vi "LSCI_6-19.vi"() -> ()   [LabVIEW 2019]
uses:
  Control 2.ctl
  Settings.ctl
  <vilib>/DAQmx/write.llb/DAQmx Write (Analog 1D DBL 1Chan NSamp).vi
  <vilib>/DAQmx/create/channels.llb/DAQmx Create Channel (AO-Voltage-Basic).vi
  <vilib>/DAQmx/configure/timing.llb/DAQmx Timing (Sample Clock).vi
  <vilib>/DAQmx/miscellaneous.llb/DAQmx Fill In Error Info.vi
panel:
  out "LSCI Sequence 2":dbl[](graph)
  in  "Stop":bool
  in  "Strength (V)":dbl=5.0
  in  "Width of pulse (ms)":dbl=70.0
  in  "Delay End (ms)":i32=52
  in  "Delay (ms)":dbl=20.0
  in  "AOM Voltage":dbl=0.135 format="%0.3f"
  out "String 7":string="AOM Settings"
  out "String 6":string="Stroke Settings"
  out "String 5":string="Intrinsic Imaging"
  in  "LED 625 nm":bool
  in  "LED 580 nm":bool
  out "Period (ms)":dbl=6.0
  out "String 4":string="Experimental Summary"
  out "String 3":string="Stimulation Control"
  out "String 2":string="Sequence Control"
  out "String":string="Trials Control"
  in  "Strength (V)":dbl=5.0
  in  "# of stimulations":i32=20
  in  "Delay (ms)":dbl=20.0
  in  "Width of pulse (ms)":dbl=70.0
  in  "# of Sequences":dbl=300.0
  in  "Delay End (ms)":i32=52
  in  "Sampling Rate (Hz)":T1=100000.0 format="%#_9f"
  in  "Frames/Seq":i32=8
  in  "Exposure Width (ms)":T1=5.0 format="%#_9f"
  in  "Time Between (ms)":T2=1.0 format="%#_9f"
  in  "Pre-stimulus Time":dbl=2.5 format="%.6f"
  in  "Time b/w Trials (s)":dbl=20.0 caption="Delay Time (s)"
  in  "# Trials":i32=50
  in  "Time domain signal":enum32{"Trigger Sequence", "Stimulation pulse"}(tab)
  out "LSCI Sequence":cluster{i32, dbl, dbl[]}(graph)={0, 1e-05, array[10000 elements]}
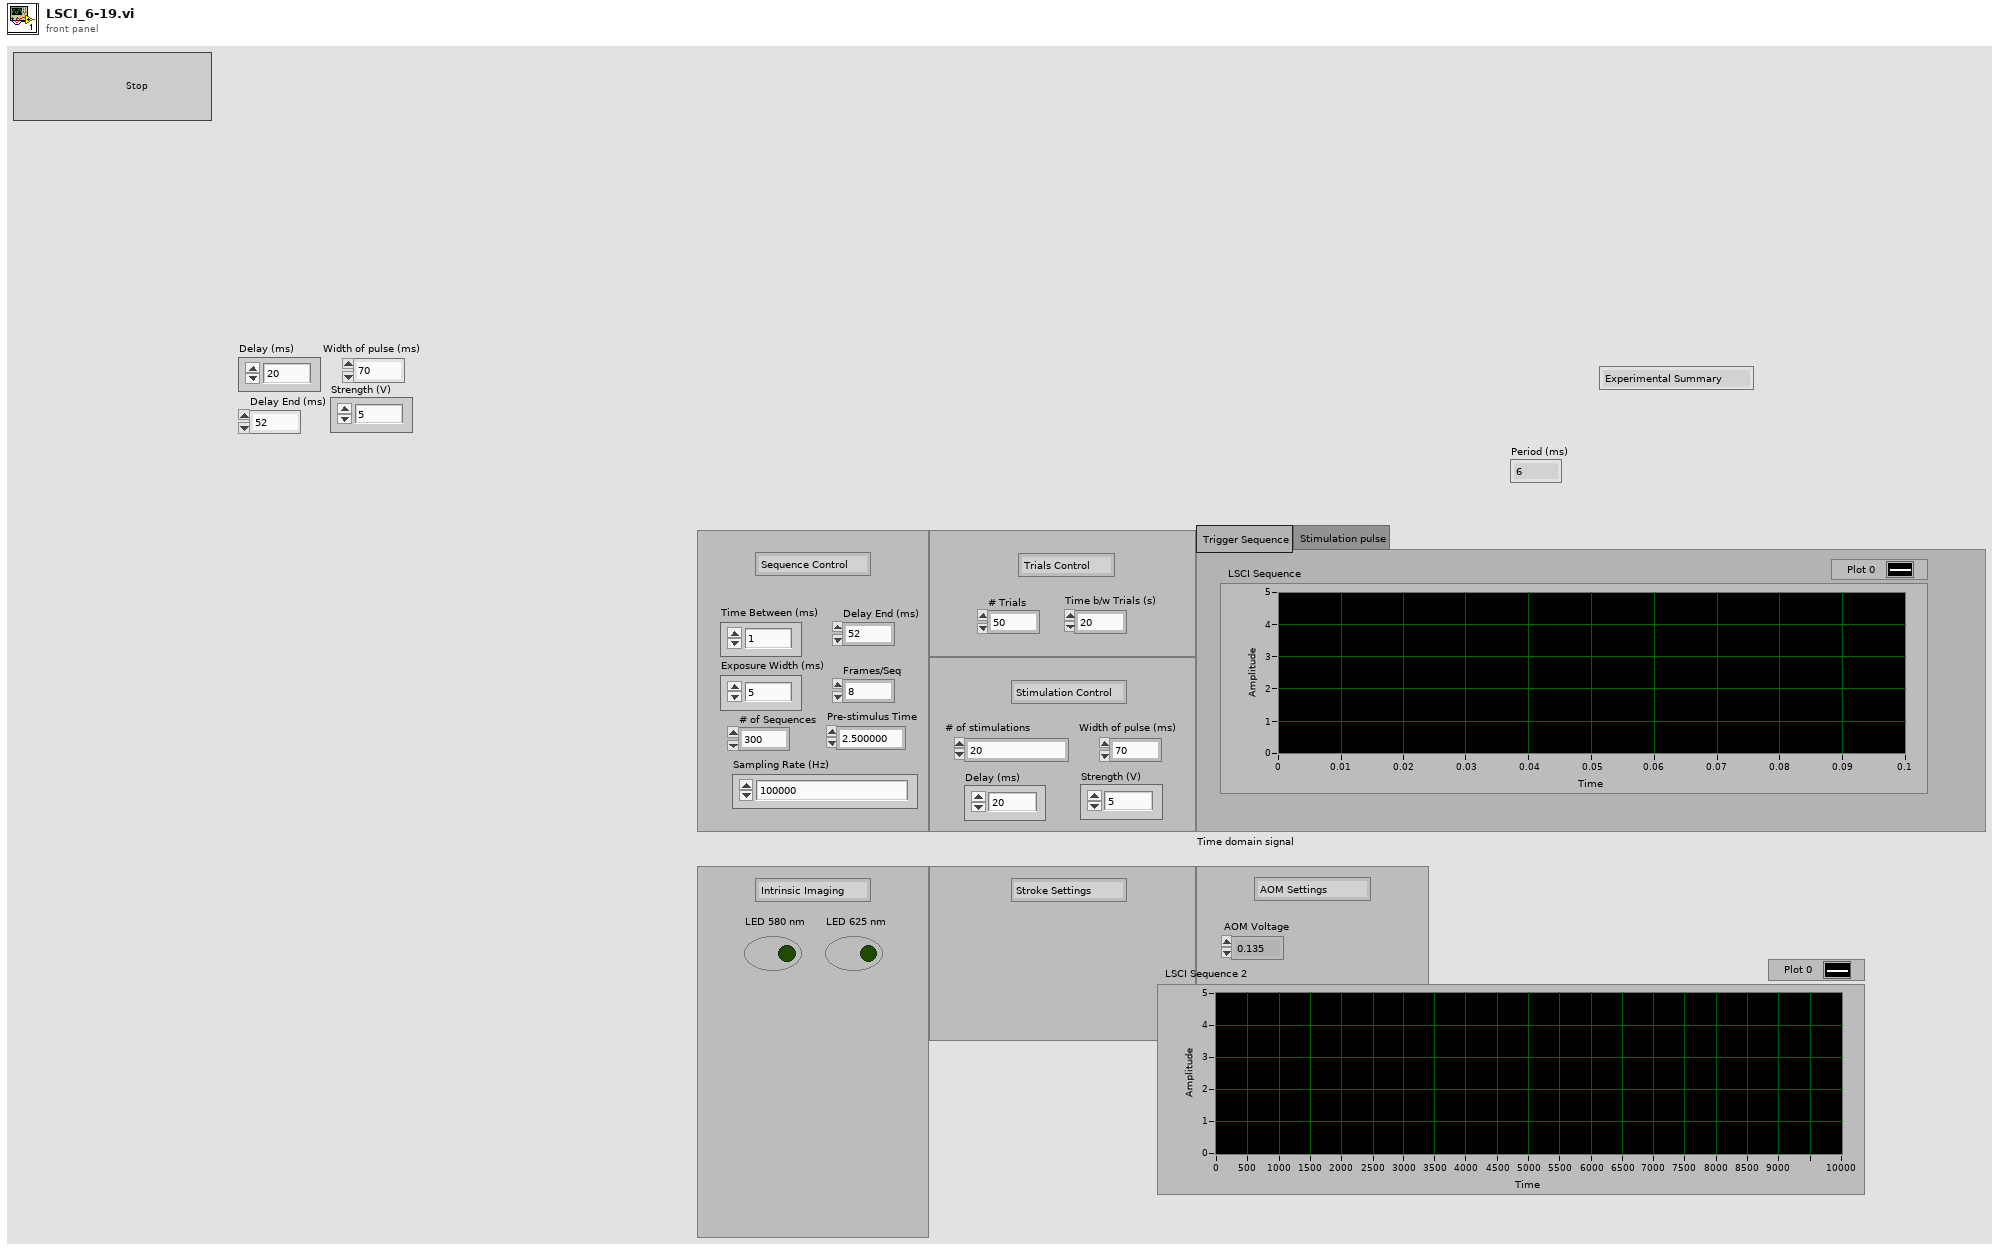
[diagram p1: front panel]
types:
  T1 = typedef "Settings.ctl" = dbl
  T2 = typedef "Control 2.ctl" = dbl
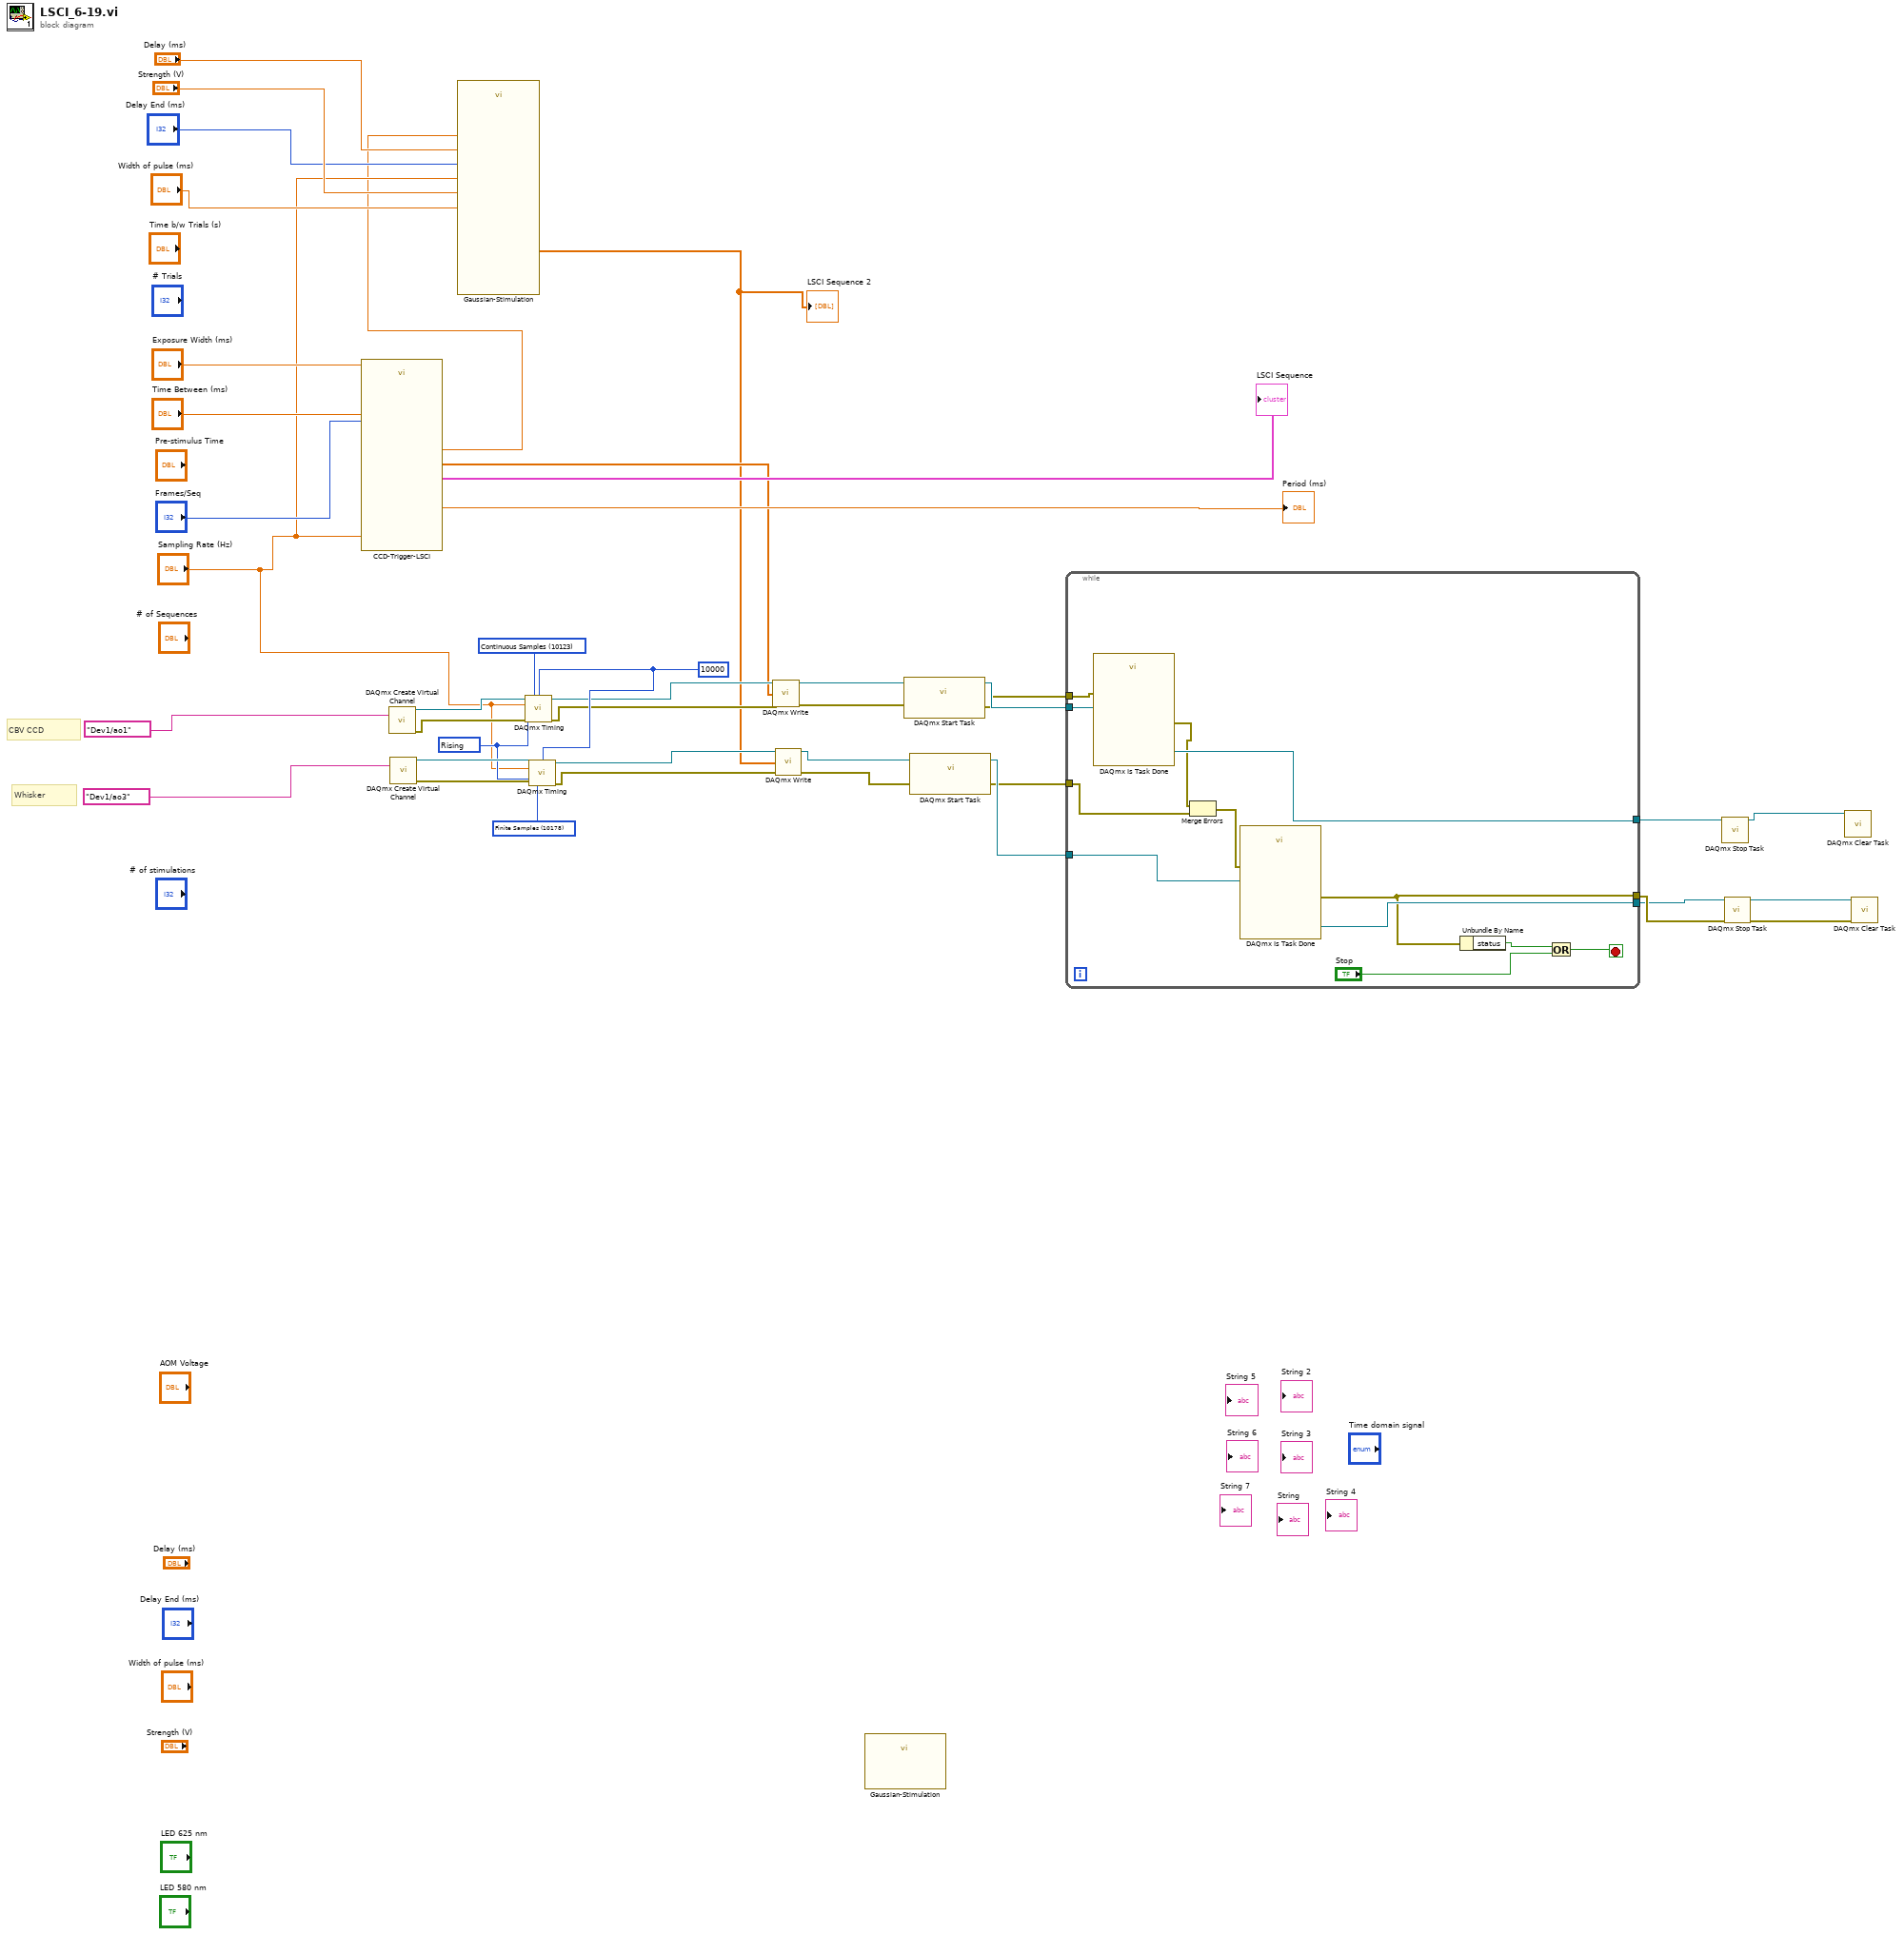
[diagram p0: block diagram]
diagram:
  w28 = 10178 items=["Finite Samples"=10178, "Continuous Samples"=10123, "Hardware Timed Single Point"=12522] ("sample mode")
  w27 = 10000 ("samples per channel")
  w32 = 10123 items=["Finite Samples"=10178, "Continuous Samples"=10123, "Hardware Timed Single Point"=12522] ("sample mode")
  w29 = 10280 items=["Rising"=10280, "Falling"=10171] ("active edge")
  # "CBV CCD"
  # "Whisker"
  n1 = call "CCD-Trigger-LSCI.vi"("Sampling Rate"="Sampling Rate (Hz)", "Time Between (ms)"="Time Between (ms)", "Exposure Width (ms) in"="Exposure Width (ms)", "Frames/Seq"="Frames/Seq") -> ("# Samples"=w2:T1, "Period (ms)"=→"Period (ms)":dbl, "Array out"=w22:dbl[], "LSCI Sequence"=→"LSCI Sequence":cluster{i32, dbl, dbl[]})  [unwired: 3 in, 1 out]
  n2 = call-poly <vilib>:"DAQmx Create Virtual Channel.vi"("physical channels"=tag "Dev1/ao1") -> ("task out"=w33:refnum<k21>, "error out"=w34:errorcluster)  [unwired: 13 in]
  n3 = call-poly <vilib>:"DAQmx Create Virtual Channel.vi"("physical channels"=tag "Dev1/ao3") -> ("task out"=w31:refnum<k21>, "error out"=w30:errorcluster)  [unwired: 13 in]
  n4 = call "Gaussian-Stimulation.vi"("Strength (V)"="Strength (V)", "Delay (ms)"="Delay (ms)", "# Samples in"=w2, "Width of pulse (ms)"="Width of pulse (ms)", "Delay End (ms)"="Delay End (ms)", "Sampling Rate"="Sampling Rate (Hz)") -> ("Array 2"=w1:T1[])  [unwired: 1 in, 4 out]
  "LSCI Sequence 2" <- w1
  n5 = call-poly <vilib>:"DAQmx Timing.vi"("task/channels in"=w33, "sample mode"=w32, "samples per channel"=w27, "rate"="Sampling Rate (Hz)", "active edge"=w29, "error in"=w34) -> ("task out"=w26:refnum<k21>, "error out"=w25:errorcluster)  [unwired: 8 in]
  n6 = call-poly <vilib>:"DAQmx Timing.vi"("task/channels in"=w31, "sample mode"=w28, "samples per channel"=w27, "rate"="Sampling Rate (Hz)", "active edge"=w29, "error in"=w30) -> ("task out"=w24:refnum<k21>, "error out"=w23:errorcluster)  [unwired: 8 in]
  n7 = call-poly <vilib>:"DAQmx Write.vi"("task/channels in"=w26, "data"=w22, "error in"=w25) -> ("task out"=w19:refnum<k21>, "error out"=w18:errorcluster)  [unwired: 10 in, 1 out]
  n8 = call-poly <vilib>:"DAQmx Write.vi"("task/channels in"=w24, "data"=w1, "error in"=w23) -> ("task out"=w21:refnum<k21>, "error out"=w20:errorcluster)  [unwired: 10 in, 1 out]
  n9 = call "Gaussian-Stimulation.vi"() -> ()  [unwired: 7 in, 5 out]
  n10 = call <vilib>:"DAQmx Start Task.vi"("task/channels in"=w19, "error in"=w18) -> ("task out"=w17:refnum<k21>, "error out"=w16:errorcluster)  [unwired: 12 in]
  n11 = call <vilib>:"DAQmx Start Task.vi"("task/channels in"=w21, "error in"=w20) -> ("task out"=w15:refnum<k21>, "error out"=w14:errorcluster)  [unwired: 12 in]
  n12 = while {
    tunnel: [w53] -> w13
    tunnel: [w52] -> w11
    tunnel: [w51] -> w12
    tunnel: w17 -> [w49]
    tunnel: w16 -> [w48]
    tunnel: w15 -> [w47]
    tunnel: w14 -> [w44]
    stop <- w50 stop-if-true
    n13 = call <vilib>:"DAQmx Is Task Done.vi"("task/channels in"=w49, "error in"=w48) -> ("task out"=w53:refnum<k21>, "error out"=w43:errorcluster)  [unwired: 11 in, 1 out]
    n14 = Merge Errors(w43, w44) -> (w42:errorcluster)
    n15 = call <vilib>:"DAQmx Is Task Done.vi"("task/channels in"=w47, "error in"=w42) -> ("task out"=w52:refnum<k21>, "error out"=w51:errorcluster)  [unwired: 11 in, 1 out]
    n16 = Unbundle By Name(w51) -> ("status"=w46:bool)
    n17 = Or(x=w46, y="Stop") -> (x .or. y?=w50:bool)
  }
  n18 = call <vilib>:"DAQmx Stop Task.vi"("task/channels in"=w13) -> ("task out"=w8:refnum<k21>)  [unwired: 13 in, 1 out]
  n19 = call <vilib>:"DAQmx Stop Task.vi"("task/channels in"=w11, "error in"=w12) -> ("task out"=w10:refnum<k21>, "error out"=w9:errorcluster)  [unwired: 12 in]
  n20 = call <vilib>:"DAQmx Clear Task.vi"("task in"=w8) -> ()  [unwired: 14 in, 1 out]
  n21 = call <vilib>:"DAQmx Clear Task.vi"("task in"=w10, "error in"=w9) -> ()  [unwired: 13 in, 1 out]
